vi "MoleculeEvap.vi"() -> ()   [LabVIEW 2020]
uses:
  <vilib>/measure/NI_MABase.lvlib
panel:
  out "Progress":u8(slide) scale=0.0..100.0
  out "Countdown":dbl
  in  "Sound":bool
  in  "Reset":bool
  in  "Startrol On":bool
  out "?":dbl format="%#.0f"
  out "?":dbl format="%#.0f"
  out "?":dbl format="%#_5g"
  out "?":dbl
  in  "A/ML":dbl
  in  "Other":bool
  in  "PTCDA":bool
  in  "Pentacene":bool
  in  "?":bool
  out "?":dbl
  out "?":dbl format="%#.0f"
  out "?":dbl
  in  "10":dbl
  in  "ML":dbl
  out "?":dbl format="%#_5g"
  out "?":dbl format="%#_5g"
  out "?":dbl
  out "?":dbl
  out "?":dbl
  out "?":dbl
  out "?":dbl
  out "?":dbl
  out "?":dbl
  out "?":dbl
  out "?":dbl
  out "?":dbl
  in  "9":dbl
  in  "8":dbl
  in  "7":dbl
  in  "6":dbl
  in  "5":dbl
  in  "4":dbl
  in  "3":dbl
  in  "2":dbl
  in  "1":dbl
  in  "0":dbl
  # "Molecule Evaporation Calculator"
  # "Calculates the time required to deposit an organic film of variable thickness, using a quartz monitor to calculate the deposition rate. \n\nNote that the simple average is calculated as the rate - dt are shown to check the rate is stable.  \n\nThe timer gives a 10 second countdown before deposition should be started & before deposition should be terminated, with a tone indicator.\n\nNo hardware is connected to this calculator."
  # "Thickness (A)"
  # "Time (min.sec)"
  # "dt (sec)"
  # "Calculations:"
  # "Thickness:"
  # "x"
  # "="
  # "A/ML"
  # "ML"
  # "A"
  # "Rate:"
  # "Molecule:"
  # "/"
  # "="
  # "sec"
  # "A"
  # "sec/A"
  # "Deposition Time:"
  # "Molecule Size:"
  # "="
  # "sec"
  # "min"
  # "sec"
  # "Coverage:"
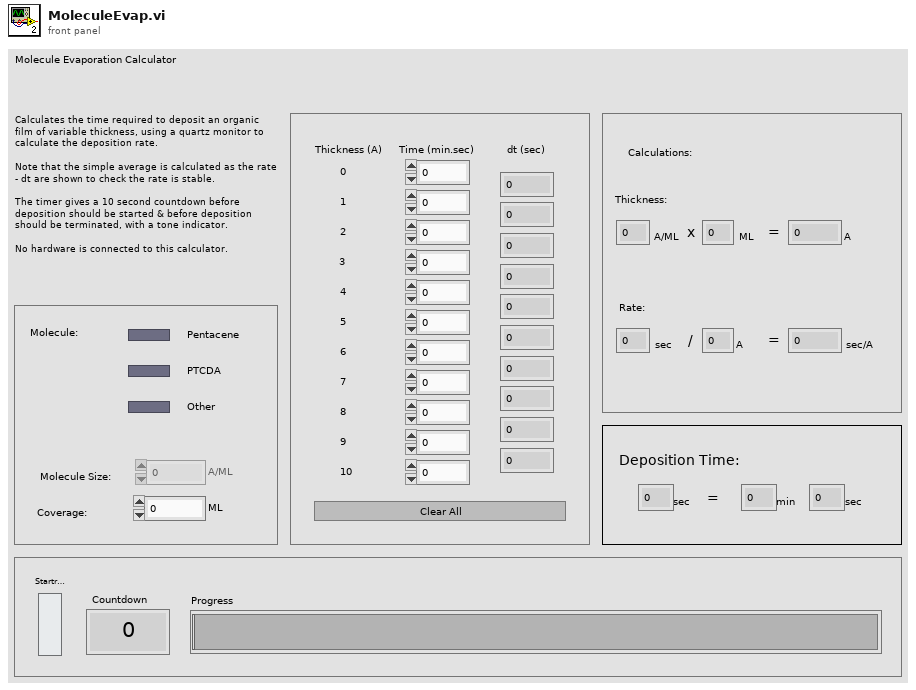
[diagram p1: front panel]
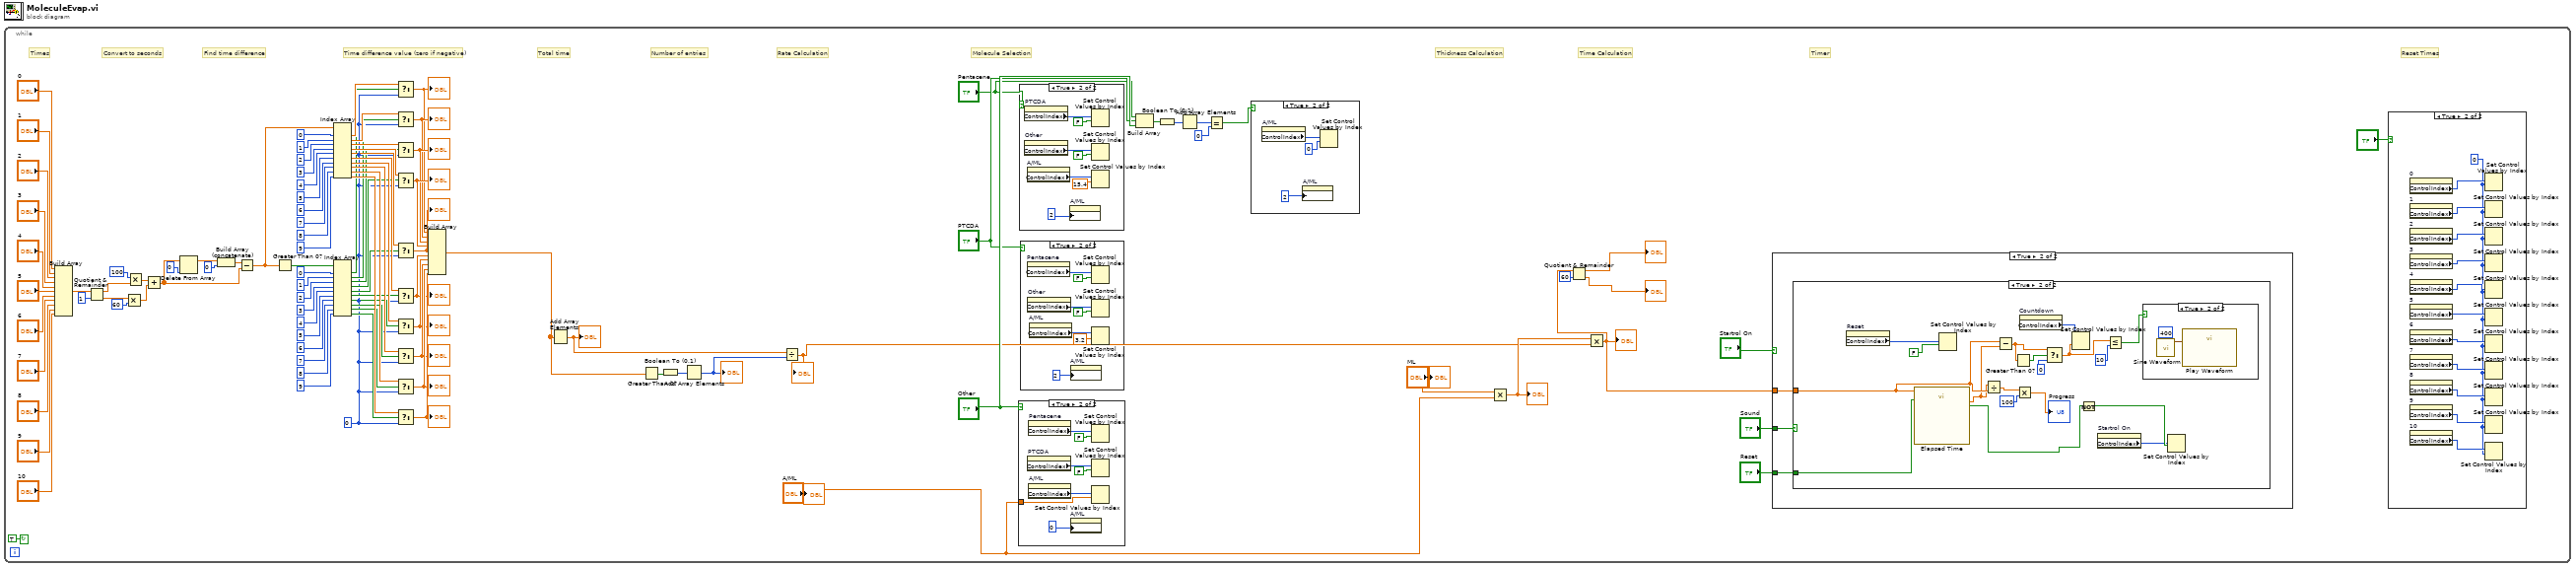
[diagram p0: block diagram]
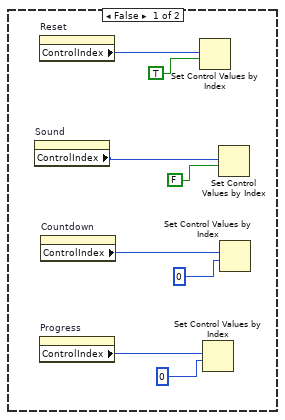
[diagram p2: hidden frame]
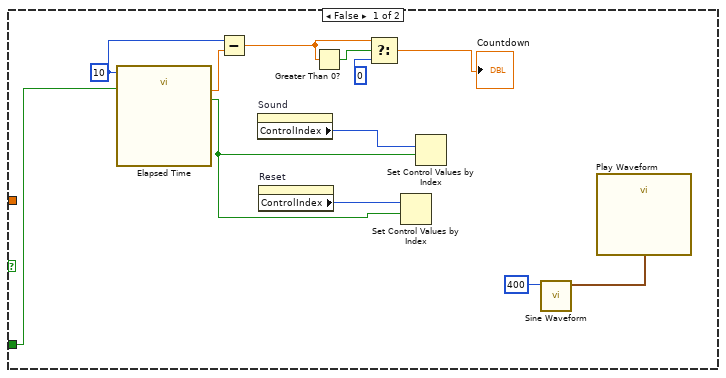
[diagram p3: hidden frame]
diagram:
  n1 = while {
    stop <- TRUE continue-if-true
    w21 = 0
    # "Timer"
    # "Reset Times"
    # "Molecule Selection"
    # "Time Calculation"
    # "Thickness Calculation"
    # "Rate Calculation"
    # "Number of entries"
    # "Total time"
    # "Time difference value (zero if negative)"
    # "Find time difference"
    # "Convert to seconds"
    # "Times"
    n2 = Build Array("0", "1", "2", "3", "4", "5", "6", "7", "8", "9", "10") -> (w49:dbl[])
    n3 = Quotient & Remainder(x=w49, y=1) -> (x-y*floor(x/y)=w48:dbl[], floor(x/y)=w45:dbl[])
    n4 = Multiply(x=w45, y=60) -> (x*y=w46:dbl[])
    n5 = Multiply(x=100, y=w48) -> (x*y=w47:dbl[])
    n6 = Add(x=w47, y=w46) -> (x+y=w72:dbl[])
    n7 = Delete From Array(array=w72, index=0) -> (array with subset deleted=w73:dbl[])  [unwired: 1 in, 1 out]
    n8 = Build Array (concatenate)(w73, 0) -> (w74:dbl[])
    n9 = Subtract(x=w74, y=w72) -> (x-y=w61:dbl[])
    n10 = Greater Than 0?(x=w61) -> (x > 0?=w50:bool[])
    n11 = Index Array(array=w61, index #1=0, index #2=1, index #3=2, index #4=3, index #5=4, index #6=5, index #7=6, index #8=7, index #9=8, index #10=9) -> (element #1=w62:dbl, element #2=w63:dbl, element #3=w64:dbl, element #4=w65:dbl, element #5=w66:dbl, element #6=w67:dbl, element #7=w68:dbl, element #8=w69:dbl, element #9=w70:dbl, element #10=w71:dbl)
    n12 = Index Array(array=w50, index #1=0, index #2=1, index #3=2, index #4=3, index #5=4, index #6=5, index #7=6, index #8=7, index #9=8, index #10=9) -> (element #1=w51:bool, element #2=w52:bool, element #3=w53:bool, element #4=w54:bool, element #5=w60:bool, element #6=w55:bool, element #7=w56:bool, element #8=w57:bool, element #9=w58:bool, element #10=w59:bool)
    n13 = Select(t=w62, s=w51, f=w21) -> (s? t:f=w75:dbl)
    "?" <- w75
    n14 = Select(t=w63, s=w52, f=w21) -> (s? t:f=w76:dbl)
    "?" <- w76
    n15 = Select(t=w64, s=w53, f=w21) -> (s? t:f=w77:dbl)
    "?" <- w77
    n16 = Select(t=w65, s=w54, f=w21) -> (s? t:f=w78:dbl)
    "?" <- w78
    n17 = Select(t=w66, s=w60, f=w21) -> (s? t:f=w79:dbl)
    "?" <- w79
    n18 = Select(t=w67, s=w55, f=w21) -> (s? t:f=w80:dbl)
    "?" <- w80
    n19 = Select(t=w68, s=w56, f=w21) -> (s? t:f=w81:dbl)
    "?" <- w81
    n20 = Select(t=w69, s=w57, f=w21) -> (s? t:f=w82:dbl)
    "?" <- w82
    n21 = Select(t=w70, s=w58, f=w21) -> (s? t:f=w83:dbl)
    "?" <- w83
    n22 = Select(t=w71, s=w59, f=w21) -> (s? t:f=w84:dbl)
    "?" <- w84
    n23 = Build Array(w75, w76, w77, w78, w79, w80, w81, w82, w83, w84) -> (w88:dbl[])
    n24 = Add Array Elements(numeric array=w88) -> (sum=w89:dbl)
    "?" <- w89
    n25 = Greater Than 0?(x=w88) -> (x > 0?=w85:bool[])
    n26 = Boolean To (0,1)(Boolean=w85) -> (0, 1=w86:i16[])
    n27 = Add Array Elements(numeric array=w86) -> (sum=w87:i16)
    "?" <- w87
    n28 = Divide(x=w89, y=w87) -> (x/y=w90:dbl)
    "?" <- w90
    n29 = case shown="True" "Other" {
      tunnel: "A/ML" -> [_ w166]
      frame False {
      }
      frame True {
        n30 = property on="PTCDA" class="Bool (strict)"() -> ("ControlIndex"=w164:i32)  [unwired: 2 in, 2 out]
        n31 = property on="Pentacene" class="Bool (strict)"() -> ("ControlIndex"=w165:i32)  [unwired: 2 in, 2 out]
        n32 = property on="A/ML" class="DigNum (strict)"() -> ("ControlIndex"=w163:i32)  [unwired: 2 in, 2 out]
        n33 = property on="A/ML" class="DigNum (strict)"("DisabledEnum"=0) -> ()  [unwired: 2 in, 2 out]
        n34 = Set Control Values by Index(1:w165, 2:FALSE) -> ()  [unwired: 2 in, 1 out]
        n35 = Set Control Values by Index(1:w164, 2:FALSE) -> ()  [unwired: 2 in, 1 out]
        n36 = Set Control Values by Index(1:w163, 2:w166) -> ()  [unwired: 2 in, 1 out]
      }
    }
    n37 = case shown="True" "Pentacene" {
      frame False {
      }
      frame True {
        n38 = property on="PTCDA" class="Bool (strict)"() -> ("ControlIndex"=w181:i32)  [unwired: 2 in, 2 out]
        n39 = property on="Other" class="Bool (strict)"() -> ("ControlIndex"=w179:i32)  [unwired: 2 in, 2 out]
        n40 = property on="A/ML" class="DigNum (strict)"() -> ("ControlIndex"=w177:i32)  [unwired: 2 in, 2 out]
        n41 = property on="A/ML" class="DigNum (strict)"("DisabledEnum"=2) -> ()  [unwired: 2 in, 2 out]
        n42 = Set Control Values by Index(1:w181, 2:FALSE) -> ()  [unwired: 2 in, 1 out]
        n43 = Set Control Values by Index(1:w179, 2:FALSE) -> ()  [unwired: 2 in, 1 out]
        n44 = Set Control Values by Index(1:w177, 2:15.4) -> ()  [unwired: 2 in, 1 out]
      }
    }
    n45 = case shown="True" "PTCDA" {
      frame False {
      }
      frame True {
        n46 = property on="Pentacene" class="Bool (strict)"() -> ("ControlIndex"=w172:i32)  [unwired: 2 in, 2 out]
        n47 = property on="Other" class="Bool (strict)"() -> ("ControlIndex"=w171:i32)  [unwired: 2 in, 2 out]
        n48 = property on="A/ML" class="DigNum (strict)"() -> ("ControlIndex"=w170:i32)  [unwired: 2 in, 2 out]
        n49 = property on="A/ML" class="DigNum (strict)"("DisabledEnum"=2) -> ()  [unwired: 2 in, 2 out]
        n50 = Set Control Values by Index(1:w172, 2:FALSE) -> ()  [unwired: 2 in, 1 out]
        n51 = Set Control Values by Index(1:w171, 2:FALSE) -> ()  [unwired: 2 in, 1 out]
        n52 = Set Control Values by Index(1:w170, 2:3.2) -> ()  [unwired: 2 in, 1 out]
      }
    }
    n53 = Build Array("Pentacene", "PTCDA", "Other") -> (w91:bool[])
    n54 = Boolean To (0,1)(Boolean=w91) -> (0, 1=w92:i16[])
    n55 = Add Array Elements(numeric array=w92) -> (sum=w96:i16)
    n56 = Equal?(x=w96, y=0) -> (x = y?=w97:bool)
    n57 = case shown="True" w97 {
      frame False {
      }
      frame True {
        n58 = property on="A/ML" class="DigNum (strict)"() -> ("ControlIndex"=w161:i32)  [unwired: 2 in, 2 out]
        n59 = property on="A/ML" class="DigNum (strict)"("DisabledEnum"=2) -> ()  [unwired: 2 in, 2 out]
        n60 = Set Control Values by Index(1:w161, 2:0) -> ()  [unwired: 2 in, 1 out]
      }
    }
    n61 = Multiply(x="ML", y="A/ML") -> (x*y=w100:dbl)
    "?" <- w100
    n62 = Multiply(x=w100, y=w90) -> (x*y=w5:dbl)
    "?" <- w5
    n63 = Quotient & Remainder(x=w5, y=60) -> (x-y*floor(x/y)=→"?":dbl, floor(x/y)=→"?":dbl)
    n64 = case shown="True" "Startrol On" {
      tunnel: w5 -> [_ w114]
      tunnel: "Reset" -> [_ w113]
      tunnel: "Sound" -> [_ w112]
      frame False {
        n65 = property on="Sound" class="Bool (strict)"() -> ("ControlIndex"=w108:i32)  [unwired: 2 in, 2 out]
        n66 = property on="Reset" class="Bool (strict)"() -> ("ControlIndex"=w111:i32)  [unwired: 2 in, 2 out]
        n67 = property on="Progress" class="Slide (strict)"() -> ("ControlIndex"=w104:i32)  [unwired: 2 in, 2 out]
        n68 = property on="Countdown" class="DigNum (strict)"() -> ("ControlIndex"=w107:i32)  [unwired: 2 in, 2 out]
        n69 = Set Control Values by Index(1:w111, 2:TRUE) -> ()  [unwired: 2 in, 1 out]
        n70 = Set Control Values by Index(1:w104, 2:0) -> ()  [unwired: 2 in, 1 out]
        n71 = Set Control Values by Index(1:w108, 2:FALSE) -> ()  [unwired: 2 in, 1 out]
        n72 = Set Control Values by Index(1:w107, 2:0) -> ()  [unwired: 2 in, 1 out]
      }
      frame True {
        n73 = case shown="True" w112 {
          tunnel: w114 -> [_ w134]
          tunnel: w113 -> [w115 w142]
          frame False {
            w123 = 10
            n74 = call "Elapsed Time"("Time Target (s)"=w123, "Reset"=w115) -> ("Elapsed Time (s)"=w122:dbl, "Time has Elapsed"=w124:bool)  [unwired: 10 in, 6 out]
            n75 = Subtract(x=w123, y=w122) -> (x-y=w117:dbl)
            n76 = property on="Sound" class="Bool (strict)"() -> ("ControlIndex"=w126:i32)  [unwired: 2 in, 2 out]
            n77 = property on="Reset" class="Bool (strict)"() -> ("ControlIndex"=w125:i32)  [unwired: 2 in, 2 out]
            n78 = Greater Than 0?(x=w117) -> (x > 0?=w118:bool)
            n79 = Select(t=w117, s=w118, f=0) -> (s? t:f=→"Countdown":dbl)
            n80 = Set Control Values by Index(1:w125, 2:w124) -> ()  [unwired: 2 in, 1 out]
            n81 = Set Control Values by Index(1:w126, 2:w124) -> ()  [unwired: 2 in, 1 out]
            n82 = call <vilib>:"Sine Waveform.vi"("frequency"=400) -> ("signal out"=w121:waveform(dbl))  [unwired: 9 in, 1 out]
            n83 = call "Play Waveform"("Data"=w121) -> ()  [unwired: 18 in, 1 out]
          }
          frame True {
            n84 = property on="Reset" class="Bool (strict)"() -> ("ControlIndex"=w139:i32)  [unwired: 2 in, 2 out]
            n85 = call "Elapsed Time"("Time Target (s)"=w134, "Reset"=w142) -> ("Elapsed Time (s)"=w133:dbl, "Time has Elapsed"=w143:bool)  [unwired: 10 in, 6 out]
            n86 = Set Control Values by Index(1:w139, 2:FALSE) -> ()  [unwired: 2 in, 1 out]
            n87 = Divide(x=w133, y=w134) -> (x/y=w138:dbl)
            n88 = Subtract(x=w134, y=w133) -> (x-y=w129:dbl)
            n89 = Greater Than 0?(x=w129) -> (x > 0?=w128:bool)
            n90 = Multiply(x=w138, y=100) -> (x*y=→"Progress":dbl)
            n91 = property on="Countdown" class="DigNum (strict)"() -> ("ControlIndex"=w135:i32)  [unwired: 2 in, 2 out]
            n92 = Select(t=w129, s=w128, f=0) -> (s? t:f=w127:dbl)
            n93 = Set Control Values by Index(1:w135, 2:w127) -> ()  [unwired: 2 in, 1 out]
            n94 = Not(x=w143) -> (.not. x?=w144:bool)
            n95 = property on="Startrol On" class="Bool (strict)"() -> ("ControlIndex"=w141:i32)  [unwired: 2 in, 2 out]
            n96 = Less Or Equal?(x=w127, y=10) -> (x <= y?=w131:bool)
            n97 = case shown="True" w131 {
              frame False {
              }
              frame True {
                n98 = call <vilib>:"Sine Waveform.vi"("frequency"=400) -> ("signal out"=w146:waveform(dbl))  [unwired: 9 in, 1 out]
                n99 = call "Play Waveform"("Data"=w146) -> ()  [unwired: 18 in, 1 out]
              }
            }
            n100 = Set Control Values by Index(1:w141, 2:w144) -> ()  [unwired: 2 in, 1 out]
          }
        }
      }
    }
    n101 = case shown="True" "?" {
      frame False {
      }
      frame True {
        w147 = 0
        n102 = property on="0" class="DigNum (strict)"() -> ("ControlIndex"=w158:i32)  [unwired: 2 in, 2 out]
        n103 = property on="1" class="DigNum (strict)"() -> ("ControlIndex"=w157:i32)  [unwired: 2 in, 2 out]
        n104 = property on="2" class="DigNum (strict)"() -> ("ControlIndex"=w156:i32)  [unwired: 2 in, 2 out]
        n105 = property on="3" class="DigNum (strict)"() -> ("ControlIndex"=w155:i32)  [unwired: 2 in, 2 out]
        n106 = property on="4" class="DigNum (strict)"() -> ("ControlIndex"=w154:i32)  [unwired: 2 in, 2 out]
        n107 = property on="5" class="DigNum (strict)"() -> ("ControlIndex"=w153:i32)  [unwired: 2 in, 2 out]
        n108 = property on="6" class="DigNum (strict)"() -> ("ControlIndex"=w152:i32)  [unwired: 2 in, 2 out]
        n109 = property on="7" class="DigNum (strict)"() -> ("ControlIndex"=w151:i32)  [unwired: 2 in, 2 out]
        n110 = property on="8" class="DigNum (strict)"() -> ("ControlIndex"=w150:i32)  [unwired: 2 in, 2 out]
        n111 = property on="9" class="DigNum (strict)"() -> ("ControlIndex"=w149:i32)  [unwired: 2 in, 2 out]
        n112 = property on="10" class="DigNum (strict)"() -> ("ControlIndex"=w148:i32)  [unwired: 2 in, 2 out]
        n113 = Set Control Values by Index(1:w158, 2:w147) -> ()  [unwired: 2 in, 1 out]
        n114 = Set Control Values by Index(1:w157, 2:w147) -> ()  [unwired: 2 in, 1 out]
        n115 = Set Control Values by Index(1:w156, 2:w147) -> ()  [unwired: 2 in, 1 out]
        n116 = Set Control Values by Index(1:w155, 2:w147) -> ()  [unwired: 2 in, 1 out]
        n117 = Set Control Values by Index(1:w154, 2:w147) -> ()  [unwired: 2 in, 1 out]
        n118 = Set Control Values by Index(1:w153, 2:w147) -> ()  [unwired: 2 in, 1 out]
        n119 = Set Control Values by Index(1:w152, 2:w147) -> ()  [unwired: 2 in, 1 out]
        n120 = Set Control Values by Index(1:w151, 2:w147) -> ()  [unwired: 2 in, 1 out]
        n121 = Set Control Values by Index(1:w150, 2:w147) -> ()  [unwired: 2 in, 1 out]
        n122 = Set Control Values by Index(1:w149, 2:w147) -> ()  [unwired: 2 in, 1 out]
        n123 = Set Control Values by Index(1:w148, 2:w147) -> ()  [unwired: 2 in, 1 out]
      }
    }
    "?" <- "ML"
    "?" <- "A/ML"
  }
